vi "PH_Sequencer.set PPMA Rods Settings.vi"(0 "i ref in":refnum<vi>, 2 "condition":T1 items=["undefined", "executing constructor", "_new: error", "_new: o.k.", "executing destructor"], 5 "error in (no error)":errorcluster) -> (14 "i ref out":refnum<vi>, 19 "error out":errorcluster)   [LabVIEW 2014, in "PH_Sequencer.lvlib"]
doc: "This VI gets whether the PPMA Rods instance is alive or not."
uses:
  PH_Sequencer.lvlib
  CS_Core/CSSystem/CSSystemLib/CSSystemLib.object condition.ctl
  CS_Core/CSSystem/CSSystemLib/CSSystemLib.lvlib
  PH_Basics/PH_Common/PH_Common.lvlib
  PH_Devices/PH_Beckhoff_PPMA-Rods/PH_Beckhoff_PPMA-Rods.lvlib
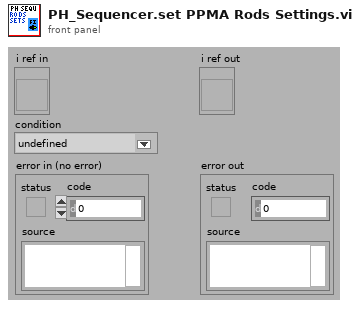
[diagram p1: front panel]
types:
  T1 = typedef "CSSystemLib.lvlib/CSSystemLib.object condition.ctl" = i32
  T2 = typedef "PH_Sequencer.lvlib/PH_Sequencer.i attribute.ctl" = cluster{"GUI Refs":cluster{"Main Off":refnum<vi>, "Fire":refnum<vi>, "Status":refnum<vi>, "Ready":refnum<vi>, "Waiting Time":refnum<vi>, "Timeout":refnum<vi>, "PPMA Ready":refnum<vi>, "Sequencer SM State":refnum<vi>, "PPPA Ready":refnum<vi>, "Calorimeter":refnum<vi>, "Beamline Ready":refnum<vi>, "Clear Beamline":refnum<vi>, "Linkage PPMA Rods":refnum<vi>, "Linkage Current PA":refnum<vi>, "Linkage Current MA":refnum<vi>, "Timing Ready":refnum<vi>, "State Timing":refnum<vi>, "Force Timing":refnum<vi>, "PSDB Shot Comment":refnum<vi>, "State PA Backreflection":refnum<vi>, "Beamline Z6 Ready":refnum<vi>, "Clear Z6 Beamline":refnum<vi>, "Sequence length":refnum<vi>, "Timing Mode":refnum<vi>, "Slow Trigger Settings":refnum<vi>, "Experiment Description":refnum<vi>, "State PSDB":refnum<vi>, "PSDB Ready":refnum<vi>, "Set PSDB Settings":refnum<vi>, "Get PSDB Info":refnum<vi>, "Take Snapshot":refnum<vi>, "Shottype":refnum<vi>, "Experiment":refnum<vi>, "Phase Frontends":refnum<vi>, "PP 45mm PILC in use":refnum<vi>}, "Status Info":cluster{"Machine Status":T3, "WaitingTime":i32, "Timeout":bool}, "Readyness":cluster{"Ready to shot":bool, "PPMA Ready":bool, "PPPA Ready":bool, "BL Ready":bool, "Timing Ready":bool, "BL Z6 Ready":bool, "PSDBReady":bool}, "Instancenames":cluster{"PPMA Rods":string, "PP Current Meas":string, "PH Beamline Chief":string, "PA Backrefl Meas":string, "Z6 Beamline Chief":string}, "Data to read":bool, "Calorimeter":cluster{"Instancename":string, "On":bool, "linked":bool}, "Linkage":cluster{"PPMA Rods":bool, "PP Current Meas":bool, "PHELIX Beamline Chief":bool, "PA Backrefl Meas":bool, "Z6 Beamline Chief":bool}, "Timing":cluster{"Instance":string, "linked":bool, "Status":T3, "Timing Mode":T4, "Slow Trigger Settings":T5, "Info available":cluster{"ext SlowTrigger":bool, "T2":bool, "Mode":bool, "Delay Slow Trigger":bool, "Phase FEs":bool}, "FE Phase":T6}, "Service ID R2S":i32, "PSDB":cluster{"Controller Instance":string, "Controller Status":T3, "Controller linked":bool, "Settings acknowledged":bool, "Current Experiment ID":i16, "Current Shot Type":i16, "Current Comment":string, "Remember Settings":bool, "Write 2 early":bool}, "PSDB Data":cluster{"Main Off?":bool, "Sequence Length":dbl, "Sequence startet":timestamp}, "6P 4Q Positions":cluster{"Instancename":string, "linked":bool, "Position":T7}[], "PUs":T8[]}
  T3 = typedef "PH_StatusHandler.lvlib/PH_StatusHandler.Status.ctl" = i16
  T4 = typedef "PH_Timing.lvlib/PH_Timing.Timing Mode.ctl" = cluster{"T2":i16, "Modeselector":enum32{"10 Hz", "0.5 Hz", "Shot"}}
  T5 = typedef "PH_Timing.lvlib/PH_Timing.Slow Trigger Settings.ctl" = cluster{"Delay":dbl, "externally triggered?":bool}
  T6 = typedef "PH_Timing.lvlib/PH_Timing.Phase FEs.ctl" = cluster{"Phase":dbl}
  T7 = typedef "PH_4_Pos_Selector.lvlib/PH_4_Pos_Selector.Position Selector.ctl" = u16
  T8 = typedef "PH_Sequencer.lvlib/PH_Sequencer.Head.ctl" = cluster{"PowerUnit":T9, "GUI Ref":refnum<vi>, "Information":T10, "linked?":bool, "GUI Ref Current Voltage":refnum<vi>}
  T9 = typedef "PH_PP_Common.lvlib/PH_PP_Common.PUs.ctl" = enum16{"no Info", "PA-19mm-1", "PA-19mm-2", "PA-45mm-PILC", "PA-45mm-MAIN", "MA-PU-1", "MA-PU-2", "MA-PU-3", "MA-PU-4", "MA-PU-5", "MA-PU-6", "MA-FR", "MA-PILC", "PA-45mm-DP"}
  T10 = typedef "PH_Sequencer.lvlib/PH_Sequencer.PU Information.ctl" = cluster{"State":T3, "Waiting Time [s]":dbl, "PU State SM":T11, "PU Timeout SM":T11}
  T11 = typedef "PH_PowerUnit_BaseClass.lvlib/PH_PowerUnit_BaseClass.SM States.ctl" = enum16{".", "Stand by", "Switch PU on", "Configure", "Set Default Voltage", "Set STANDBY", "Set READY", "Wait for Shot Cmd", "Open Dump Rods", "Open Ross Relais", "Close Ross Relais", "Switch PSU on", "Switch PSU off", "Charge", "Switch GD Channel on", "Close Dump Rods", "Rods-TO", "RR-TO", "PSU-TO", "Trigger-TO"}
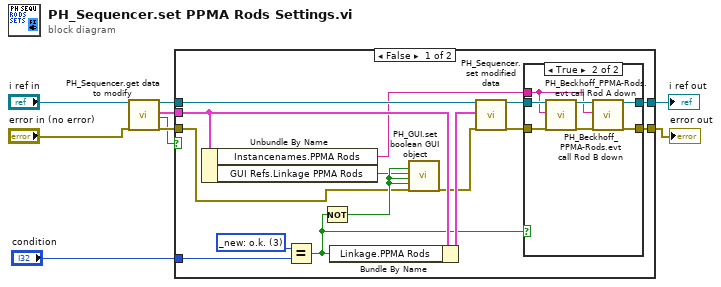
[diagram p0: block diagram]
diagram:
  n1 = call "PH_Sequencer.get data to modify.vi"("i ref in"="i ref in", "error in (no error)"="error in (no error)") -> ("i ref out"=w7:refnum<vi>, "i attribute"=w9:T2, "timed out"=w4:bool, "error out"=w5:errorcluster)  [unwired: 14 in]
  n2 = case shown="False" w4 {
    tunnel: w7 -> [w20 w35]
    tunnel: [w11 w35] -> w3
    tunnel: w5 -> [w16 w34]
    tunnel: [w10 w34] -> w2
    tunnel: w9 -> [w24 _]
    tunnel: "condition" -> [w13 _]
    frame False {
      w12 = T1 3 items=["undefined", "executing constructor", "_new: error", "_new: o.k.", "executing destructor"] ("y")
      n3 = Unbundle By Name(w24) -> ("Instancenames.PPMA Rods"=w19:string, "GUI Refs.Linkage PPMA Rods"=w14:refnum<vi>)
      n4 = Equal?(x=w12, y=w13) -> (x = y?=w15:bool)
      n5 = Not(x=w15) -> (.not. x?=w18:bool)
      n6 = Bundle By Name(cluster=w24, "Linkage.PPMA Rods"=w15) -> (w23:T2)
      n7 = call "PH_GUI.set boolean GUI object.vi"("Visible (true)"=w18, "Boolean Knob GUI Ref"=w14, "Value"=w18, "Blinking? (false)"=w18, "error in (no error)"=w16) -> ("error out"=w17:errorcluster)  [unwired: 14 in]
      n8 = call "PH_Sequencer.set modified data.vi"("i ref in"=w20, "i attribute"=w23, "error in (no error)"=w17) -> ("i ref out"=w22:refnum<vi>, "error out"=w21:errorcluster)  [unwired: 15 in]
      n9 = case shown="True" w15 {
        tunnel: w22 -> [w25 w32]
        tunnel: [w25 w28] -> w11
        tunnel: w21 -> [w26 w33]
        tunnel: [w26 w31] -> w10
        tunnel: w19 -> [_ w27]
        frame False {
        }
        frame True {
          n10 = call "PH_Beckhoff_PPMA-Rods.evt call Rod A down.vi"("i ref in"=w32, "Instance name"=w27, "error in"=w33) -> ("i ref out"=w29:refnum<vi>, "error out"=w30:errorcluster)  [unwired: 15 in]
          n11 = call "PH_Beckhoff_PPMA-Rods.evt call Rod B down.vi"("i ref in"=w29, "Instance name"=w27, "error in"=w30) -> ("i ref out"=w28:refnum<vi>, "error out"=w31:errorcluster)  [unwired: 15 in]
        }
      }
    }
    frame True {
    }
  }
  "i ref out" <- w3
  "error out" <- w2
